vi "WriteHelper.vi"(0 "object in":refnum<class "Experiment.lvclass">, 1 "Group name":string, 2 "Channel Names":string[](array[string]), 3 "Data array":sgl[](array[numeric]), 5 "error in (no error)":errorcluster) -> (14 "object out":refnum<class "Experiment.lvclass">, 19 "error out":errorcluster)   [LabVIEW 2021, in "Experiment.lvclass"]
uses:
  Experiment.lvclass
  Experiment.lvclass/Experiment.ctl
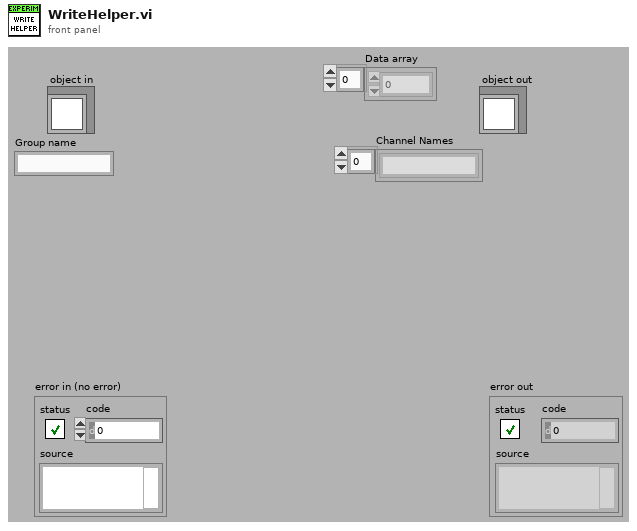
[diagram p1: front panel]
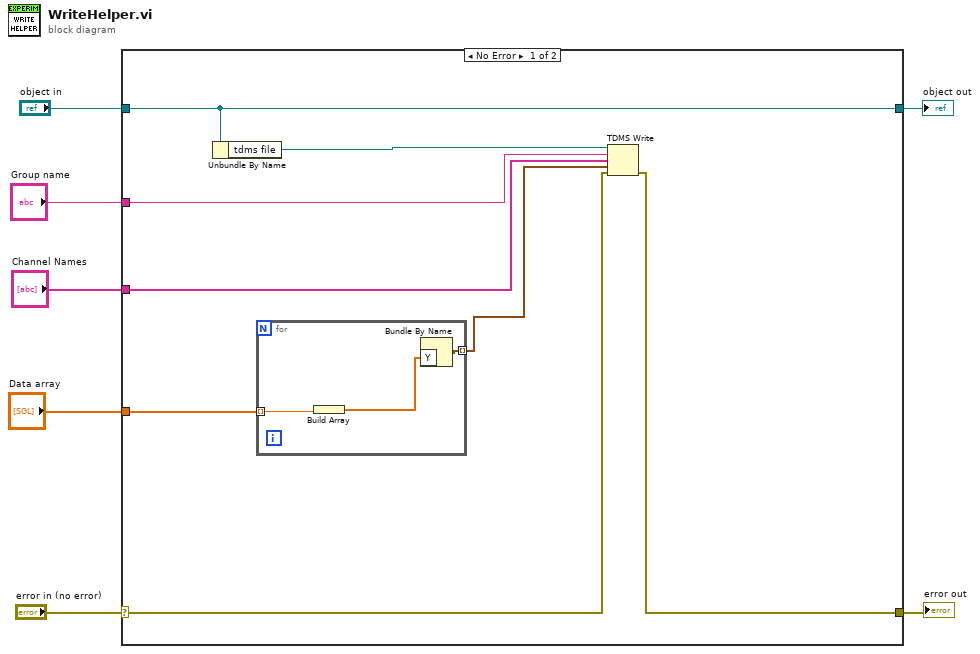
[diagram p0: block diagram]
diagram:
  n1 = case shown="No Error" "error in (no error)" {
    selector: "error in (no error)" -> [w9 w20]
    tunnel: [w8 w20] -> w6
    tunnel: [w15 w19] -> w4
    tunnel: "object in" -> [w15 w19]
    tunnel: "Data array" -> [w13 _]
    tunnel: "Channel Names" -> [w11 _]
    tunnel: "Group name" -> [w10 _]
    frame No Error {
      n2 = Unbundle By Name(w15) -> ("tdms file"=w14:refnum<k34>)
      n3 = for {
        tunnel: [w18] -> w12 mode=indexing
        tunnel: w13 -> [w17] mode=indexing
        n4 = Build Array(w17) -> (w16:sgl[])
        n5 = Bundle By Name("Y"=w16) -> (w18:waveform(sgl))  [unwired: 1 in]
      }
      n6 = TDMS Write(0:w14, 5:w10, 7:w11, 9:w12, 11:w9) -> (15:w8:errorcluster)  [unwired: 1 in, 3 out]
    }
    frame Error {
    }
  }
  "error out" <- w6
  "object out" <- w4
